vi "2-2-4 LV Timestamp to UNIX Timestamp.vi"() -> ()   [LabVIEW 2020]
panel:
  out "UNIX Timestamp":i64
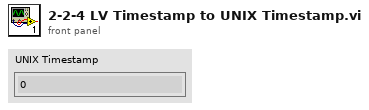
[diagram p1: front panel]
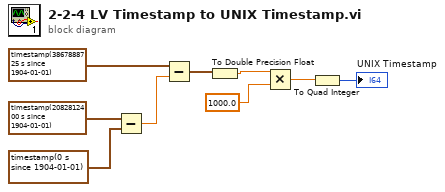
[diagram p0: block diagram]
diagram:
  n1 = Subtract(x=timestamp(2082812400 s since 1904-01-01), y=timestamp(0 s since 1904-01-01)) -> (x-y=w3:dbl)
  n2 = Subtract(x=timestamp(3867888725 s since 1904-01-01), y=w3) -> (x-y=w2:timestamp)
  n3 = To Double Precision Float(number=w2) -> (double precision float=w1:dbl)
  n4 = Multiply(x=w1, y=1000.0) -> (x*y=w8:dbl)
  n5 = To Quad Integer(1:w8) -> (0:→"UNIX Timestamp":i64)
